vi "Write Visa com port.vi"(8 "error in (no error)":errorcluster, 10 "Visa com port":string, 11 "Serial device in":refnum<class "Serial device.lvclass">) -> (0 "error out":errorcluster, 3 "Serial device out":refnum<class "Serial device.lvclass">)   [LabVIEW 2020, in "Serial device.lvclass"]
uses:
  Serial device.lvclass
  Serial device.lvclass/Serial device.ctl
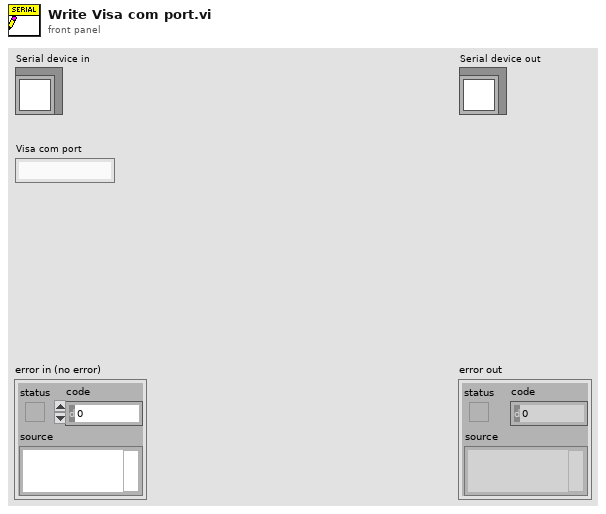
[diagram p1: front panel]
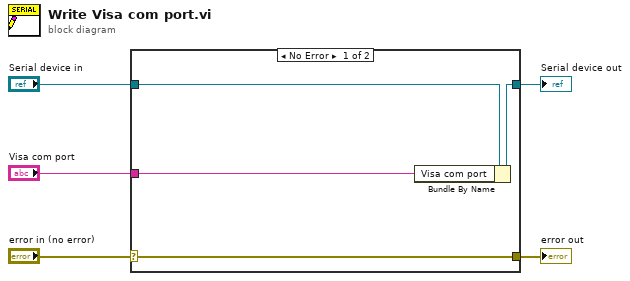
[diagram p0: block diagram]
diagram:
  n1 = case shown="No Error" "error in (no error)" {
    selector: "error in (no error)" -> [w9 w10]
    tunnel: [w9 w10] -> w4
    tunnel: [w7 w11] -> w2
    tunnel: "Serial device in" -> [w8 w11]
    tunnel: "Visa com port" -> [w6 _]
    frame No Error {
      n2 = Bundle By Name(cluster=w8, "Visa com port"=w6) -> (w7:refnum<class "Serial device.lvclass">)
    }
    frame Error {
    }
  }
  "error out" <- w4
  "Serial device out" <- w2
